vi "Play.vi"(8 "error in (no error)":errorcluster, 9 "fileName":string, 10 "audioType":string, 11 "AudioPlayer in":refnum<class "AudioPlayer.lvclass">) -> (0 "error out":errorcluster, 3 "AudioPlayer out":refnum<class "AudioPlayer.lvclass">)   [LabVIEW 2017, in "AudioPlayer.lvclass"]
uses:
  AudioPlayer.lvclass
  AudioPlayer.lvclass/AudioPlayer.ctl
  Media Adapter/MediaAdapter.lvclass
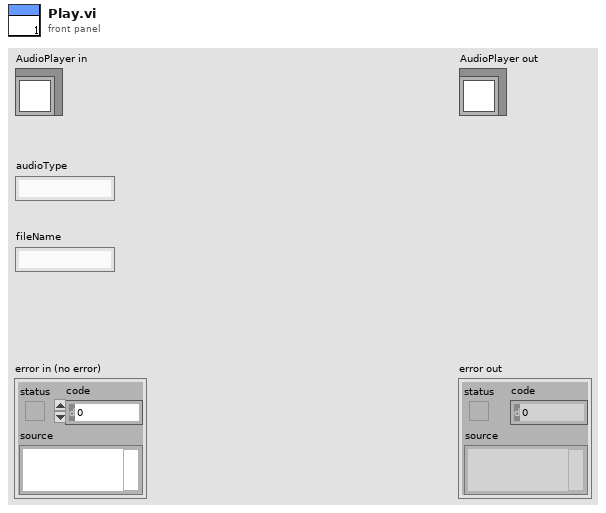
[diagram p1: front panel]
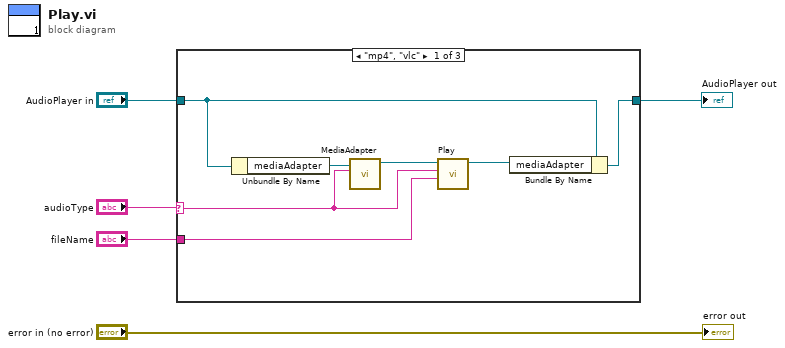
[diagram p0: block diagram]
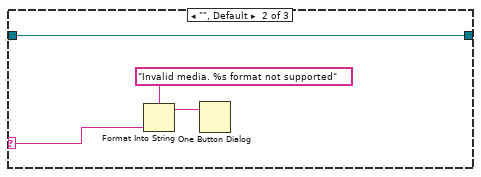
[diagram p2: hidden frame]
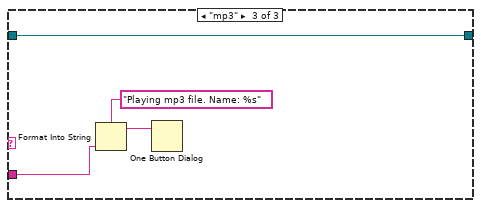
[diagram p3: hidden frame]
diagram:
  n1 = case shown="\"mp4\", \"vlc\"" "audioType" {
    selector: "audioType" -> [w6 w13 _]
    tunnel: [w10 w16 w20] -> w4
    tunnel: "AudioPlayer in" -> [w12 w16 w20]
    tunnel: "fileName" -> [w7 _ w17]
    frame "mp4", "vlc" {
      n2 = Unbundle By Name(w12) -> ("mediaAdapter"=w11:refnum<class "MediaAdapter.lvclass">)
      n3 = call "MediaAdapter.vi"("audioType"=w6, "MediaAdapter in"=w11) -> ("MediaAdapter out"=w9:refnum<class "MediaAdapter.lvclass">)  [unwired: 8 in, 1 out]
      n4 = call-dynamic "Play.vi"("fileName"=w7, "audioType"=w6, "MediaAdapter in"=w9) -> ("MediaAdapter out"=w8:refnum<class "MediaAdapter.lvclass">)  [unwired: 7 in, 1 out]
      n5 = Bundle By Name(cluster=w12, "mediaAdapter"=w8) -> (w10:refnum<class "AudioPlayer.lvclass">)
    }
    frame "", Default {
      n6 = Format Into String(format string="Invalid media. %s format not supported", w13) -> (resulting string=w15:string)  [unwired: 2 in, 1 out]
      n7 = One Button Dialog(message=w15) -> ()  [unwired: 1 in, 1 out]
    }
    frame "mp3" {
      n8 = Format Into String(format string="Playing mp3 file. Name: %s", w17) -> (resulting string=w19:string)  [unwired: 2 in, 1 out]
      n9 = One Button Dialog(message=w19) -> ()  [unwired: 1 in, 1 out]
    }
  }
  "AudioPlayer out" <- w4
  "error out" <- "error in (no error)"
